vi "PV Example Test Parameter.vi"(7 "Adress of unit":u16=1 min=1 max=255 step=1, 8 "Data":string="=?", 9 "Parameter\nread only<->describe":bool, 10 "Parameter-number":u16=315 min=1 max=999 step=1, 11 "COM Port Name in":refnum<visa-resource-name>="COM1") -> (4 "response (data)":string)   [LabVIEW 2016, in "Pfeiffer Vacuum.lvlib"]
doc: "This VI is an example of how to use the Pfeiffer Vacuum subVIs programmatically. This VI first initializes the instrument, takes measurements, then closes the instrument.\n\nWARNINGS: \nYou MUST have VISA Version 2.0 or higher installed to use this Instrument driver."
uses:
  Pfeiffer Vacuum.lvlib
panel:
  out "error out":errorcluster
  in  "error in (no error)":errorcluster
  in  "Data Typ in":string="1"
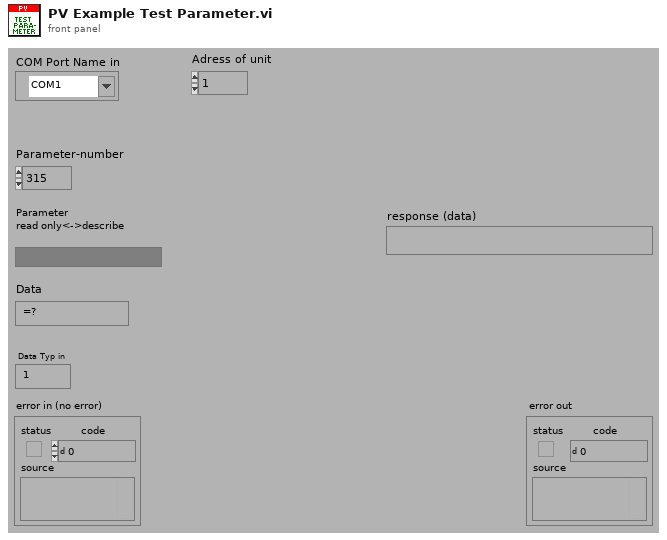
[diagram p1: front panel]
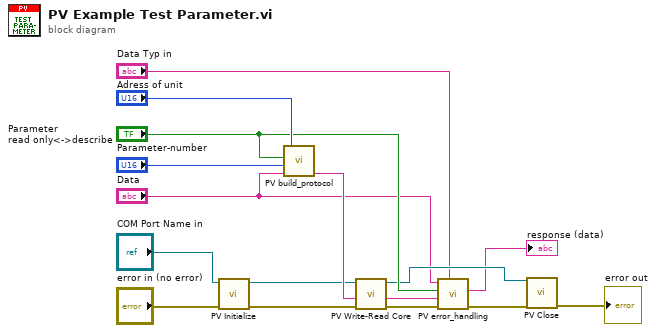
[diagram p0: block diagram]
diagram:
  n1 = call "PV Initialize.vi"("error in (no error)"="error in (no error)", "VISA session in"="COM Port Name in") -> ("error out"=w5:errorcluster, "VISA session out"=w6:refnum<visa-resource-name>)  [unwired: 8 in]
  n2 = call "PV build_protocol.vi"("Data"="Data", "Parameter-number"="Parameter-number", "parameter\nread<->describe"="Parameter\nread only<->describe", "Adress"="Adress of unit") -> ("output"=w15:string)  [unwired: 3 in]
  n3 = call "PV Write-Read Core.vi"("error in"=w5, "Write data in"=w15, "VISA session"=w6) -> ("error out"=w12:errorcluster, "response (data) out"=w13:string, "dup VISA session"=w10:refnum<visa-resource-name>)  [unwired: 2 in]
  n4 = call "PV error_handling.vi"("Data Typ in"="Data Typ in", "error in"=w12, "response (data) in"=w13, "Parameter\nread only<->describe"="Parameter\nread only<->describe", "data in"="Data") -> ("error out"=w11:errorcluster, "Data out"=→"response (data)":string)  [unwired: 4 in, 1 out]
  n5 = call "PV Close.vi"("VISA session"=w10, "error in (no error)"=w11) -> ("error out"=→"error out":errorcluster)  [unwired: 13 in]
